vi "Newmark-Status-All.vi"(0 "Table VRN IN":refnum<visa-resource-name>="COM10", 1 "Bool Refnum":refnum<vi>, 4 "StageTag":string[](array[string])=["AX", "AY", "AZ"], 5 "Error IN":errorcluster) -> (6 "?AC":dbl[](array[numeric]) format="%#.6f", 7 "?ES":i32[](array[numeric]), 8 "?VB":dbl[](array[numeric]), 9 "?LS":string[](array[string]), 10 "?VL":dbl[](array[numeric]), 11 "?SL":string[](array[string]), 12 "?UU":dbl[](array[numeric]), 13 "?TL":string[](array[string]), 14 "Table VRN OUT":refnum<visa-resource-name>="COM10", 16 "?ER":dbl[](array[numeric]) format="%.6g", 17 "?EH":string[](array[string]), 18 "Exception":string, 19 "Error OUT":errorcluster)   [LabVIEW 2011]
uses:
  Comm/SerialCommError.vi
panel:
  out "n_found":i32[](array[numeric])
  out "Error?":bool=TRUE
  out "?DB (normalized?)":bool[](array[boolean])
  out "array":string[](array[string])
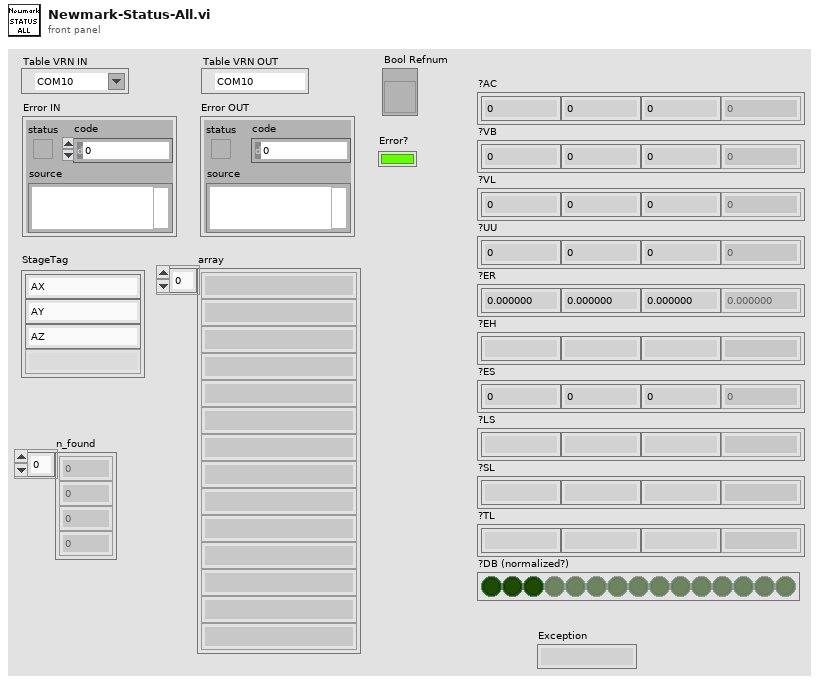
[diagram p1: front panel]
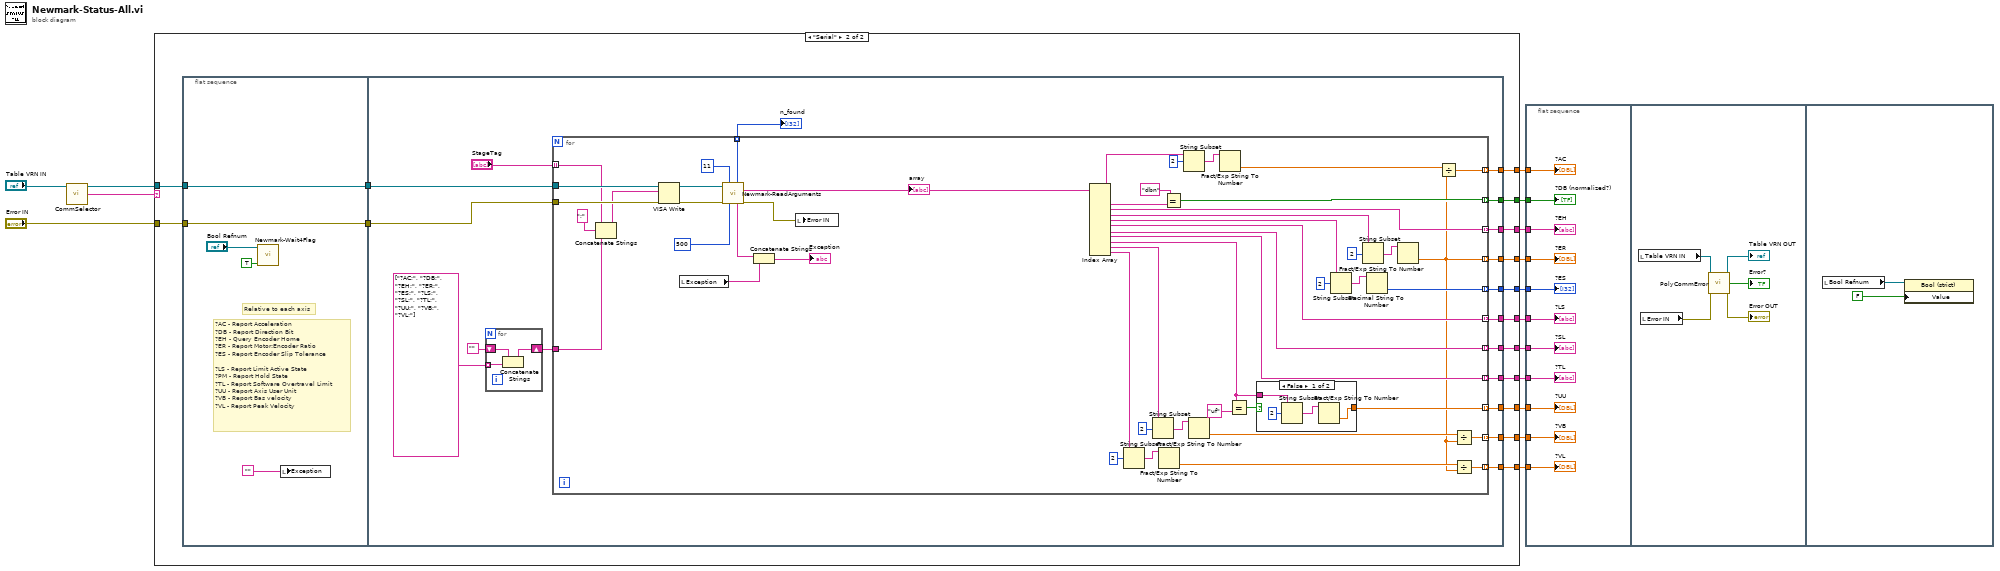
[diagram p0: block diagram]
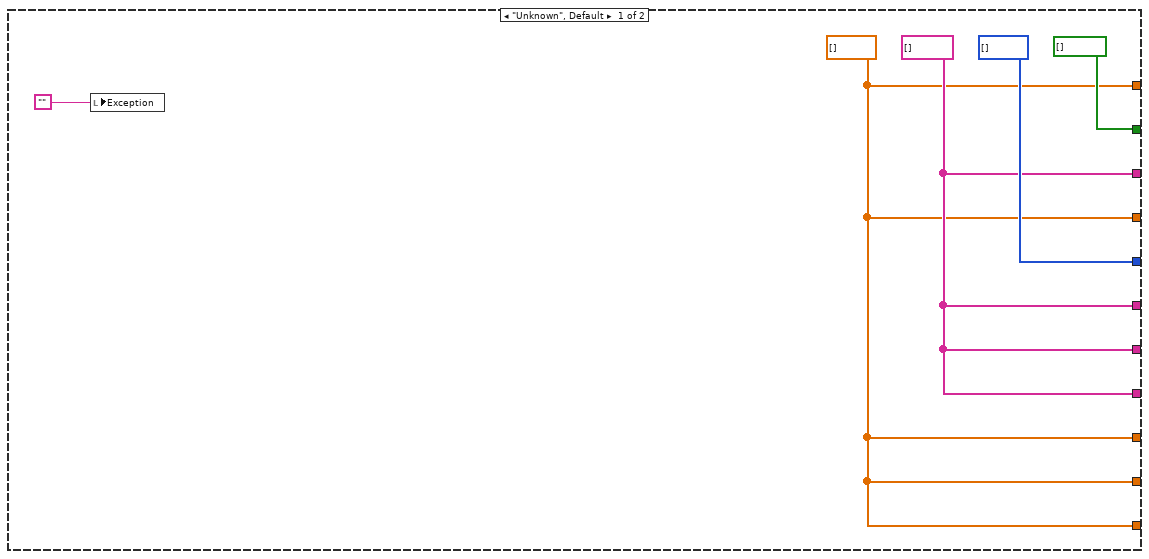
[diagram p2: hidden frame]
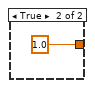
[diagram p3: hidden frame]
diagram:
  n1 = call "CommSelector.vi"("VISA resource name"="Table VRN IN") -> ("VISA resource name"=w2:refnum<visa-resource-name>, "CommType"=w1:string)  [unwired: 13 in]
  n2 = case shown="\"Serial\"" w1 {
    tunnel: "Error IN" -> [_ w33]
    tunnel: [w17 w32] -> w14
    tunnel: [bool[] [] w31] -> w13
    tunnel: [w18 w30] -> w12
    tunnel: [w17 w29] -> w11
    tunnel: [i32[] [] w28] -> w10
    tunnel: [w18 w27] -> w9
    tunnel: [w18 w26] -> w8
    tunnel: [w18 w25] -> w7
    tunnel: [w17 w24] -> w6
    tunnel: [w17 w23] -> w5
    tunnel: [w17 w22] -> w4
    tunnel: w2 -> [_ w21]
    frame "Unknown", Default {
      w18 = string[] []
      w17 = dbl[] []
      n3 = local write "Exception"("" ("Exception")) -> ()
    }
    frame "Serial" {
      n4 = flat-sequence {
        tunnel: w33 -> [w40]
        tunnel: [w36] -> w35
        tunnel: [w40] -> w34
        tunnel: w21 -> [w36]
        tunnel: [w56] -> w32
        tunnel: [w55] -> w31
        tunnel: [w54] -> w30
        tunnel: [w53] -> w29
        tunnel: [w52] -> w28
        tunnel: [w51] -> w27
        tunnel: [w50] -> w26
        tunnel: [w49] -> w25
        tunnel: [w48] -> w24
        tunnel: [w47] -> w23
        tunnel: [w46] -> w22
        tunnel: w35 -> [w58]
        tunnel: w34 -> [w57]
        frame #0 {
          # "Relative to each axis"
          # "?AC - Report Acceleration\n?DB - Report Direction Bit\n?EH - Query Encoder Home\n?ER - Report Motor:Encoder Ratio\n?ES - Report Encoder Slip Tolerance\n\n?LS - Report Limit Active State\n?PM - Report Hold State\n?TL - Report Software Overtravel Limit\n?UU - Report Axis User Unit\n?VB - Report Bas velocity\n?VL - Report Peak Velocity"
          n5 = call "Newmark-Wait4Flag.vi"("Raise Flag ?"=TRUE, "Ctl Refnum IN"="Bool Refnum") -> ()  [unwired: 8 in, 2 out]
          n6 = local write "Exception"("" ("Exception")) -> ()
        }
        frame #1 {
          n7 = for {
            shift-right: [w60] -> w42
            shift-left: "" -> [w61]
            tunnel: string[] ["?AC;", "?DB;", "?EH;", "?ER;", "?ES;", "?LS;", "?SL;", "?TL;", "?UU;", "?VB;", "?VL;"] -> [w59] mode=indexing
            n8 = Concatenate Strings(w61, w59) -> (w60:string)
          }
          n9 = for {
            tunnel: "StageTag" -> [w109] mode=indexing
            tunnel: w58 -> [w110]
            tunnel: w57 -> [w111]
            tunnel: w42 -> [w107]
            tunnel: [w78] -> w56 mode=indexing
            tunnel: [w100] -> w55 mode=indexing
            tunnel: [w99] -> w54 mode=indexing
            tunnel: [w72] -> w53 mode=indexing
            tunnel: [w92] -> w52 mode=indexing
            tunnel: [w91] -> w51 mode=indexing
            tunnel: [w90] -> w50 mode=indexing
            tunnel: [w89] -> w49 mode=indexing
            tunnel: [w85] -> w48 mode=indexing
            tunnel: [w75] -> w47 mode=indexing
            tunnel: [w76] -> w46 mode=indexing
            tunnel: [w66] -> w41 mode=indexing
            n10 = Concatenate Strings(w109, ";" ("string"), w107) -> (w106:string)
            n11 = VISA Write(VISA resource name=w110, write buffer=w106, error in (no error)=w111) -> (VISA resource name out=w71:refnum<visa-resource-name>, error out=w70:errorcluster)  [unwired: 1 out]
            n12 = local read "Exception"() -> (w64:string)
            n13 = call "Newmark-ReadArguments.vi"("Table VRN IN"=w71, "N_Args"=11, "Error IN"=w70, "Timeout (ms)"=u32 500) -> ("N_Found"=w66:i32, "Args"=w67:string[], "Exception"=w63:string, "Error OUT"=w65:errorcluster)  [unwired: 6 in, 2 out]
            "array" <- w67
            n14 = Concatenate Strings(w63, w64) -> (→"Exception":string)
            n15 = local write "Error IN"(w65) -> ()
            n16 = Index Array(array=w67) -> (element #1=w105:string, element #2=w102:string, element #3=w99:string, element #4=w96:string, element #5=w93:string, element #6=w91:string, element #7=w90:string, element #8=w89:string, element #9=w86:string, element #10=w80:string, element #11=w79:string)  [unwired: 11 in]
            n17 = String Subset(string=w79, offset (0)=2) -> (substring=w82:string)  [unwired: 1 in]
            n18 = String Subset(string=w80, offset (0)=2) -> (substring=w83:string)  [unwired: 1 in]
            n19 = Fract/Exp String To Number(string=w82) -> (number=w74:dbl)  [unwired: 3 in, 1 out]
            n20 = Equal?(x="dbn", y=w102) -> (x = y?=w100:bool)
            n21 = String Subset(string=w105, offset (0)=2) -> (substring=w103:string)  [unwired: 1 in]
            n22 = Fract/Exp String To Number(string=w83) -> (number=w73:dbl)  [unwired: 3 in, 1 out]
            n23 = Fract/Exp String To Number(string=w103) -> (number=w77:dbl)  [unwired: 3 in, 1 out]
            n24 = Equal?(x=w86, y="uf") -> (x = y?=w87:bool)
            n25 = case shown="False" w87 {
              tunnel: w86 -> [w115 _]
              tunnel: [w112 1.0] -> w85
              frame False {
                n26 = String Subset(string=w115, offset (0)=2) -> (substring=w113:string)  [unwired: 1 in]
                n27 = Fract/Exp String To Number(string=w113) -> (number=w112:dbl)  [unwired: 3 in, 1 out]
              }
              frame True {
              }
            }
            n28 = String Subset(string=w93, offset (0)=2) -> (substring=w95:string)  [unwired: 1 in]
            n29 = String Subset(string=w96, offset (0)=2) -> (substring=w98:string)  [unwired: 1 in]
            n30 = Decimal String To Number(string=w95) -> (number=w92:i32)  [unwired: 2 in, 1 out]
            n31 = Fract/Exp String To Number(string=w98) -> (number=w72:dbl)  [unwired: 3 in, 1 out]
            n32 = Divide(x=w77, y=w72) -> (x/y=w78:dbl)
            n33 = Divide(x=w73, y=w72) -> (x/y=w75:dbl)
            n34 = Divide(x=w74, y=w72) -> (x/y=w76:dbl)
          }
          "n_found" <- w41
        }
      }
    }
  }
  n35 = flat-sequence {
    tunnel: w14 -> [w127]
    tunnel: w13 -> [w126]
    tunnel: w12 -> [w125]
    tunnel: w11 -> [w124]
    tunnel: w10 -> [w123]
    tunnel: w9 -> [w122]
    tunnel: w8 -> [w121]
    tunnel: w7 -> [w120]
    tunnel: w6 -> [w119]
    tunnel: w5 -> [w118]
    tunnel: w4 -> [w117]
    frame #0 {
      "?AC" <- w127
      "?DB (normalized?)" <- w126
      "?EH" <- w125
      "?ER" <- w124
      "?ES" <- w123
      "?LS" <- w122
      "?SL" <- w121
      "?TL" <- w120
      "?UU" <- w119
      "?VB" <- w118
      "?VL" <- w117
    }
    frame #1 {
      n36 = local read "Table VRN IN"() -> (w129:refnum<visa-resource-name>)
      n37 = local read "Error IN"() -> (w130:errorcluster)
      n38 = call-poly "PolyCommError.vi"("VISA IN"=w129, "error IN"=w130) -> ("VISA OUT"=→"Table VRN OUT":refnum<visa-resource-name>, "Error"=→"Error?":bool, "error OUT"=→"Error OUT":errorcluster)  [unwired: 11 in]
    }
    frame #2 {
      n39 = local read "Bool Refnum"() -> (w133:refnum<vi>)
      n40 = property class="Bool (strict)"(reference=w133, "Value"=FALSE) -> ()  [unwired: 1 in, 2 out]
    }
  }
